vi "停止.vi"(6 "AxisHandle_Array":u32[](array[numeric]), 7 "索引":i32, 9 "停止模式":enum32{"Dec", "Emg"}(radio), 10 "reference输入":refnum<vi>, 11 "Boolean输入":refnum<vi>) -> (2 "急速停止成功":bool, 3 "减速停止成功":bool)   [LabVIEW 2016]
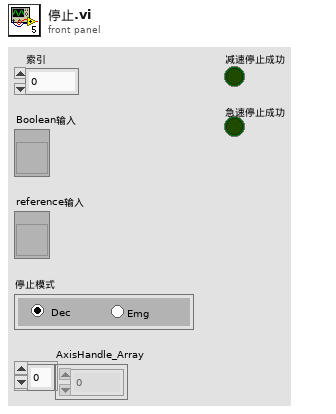
[diagram p1: front panel]
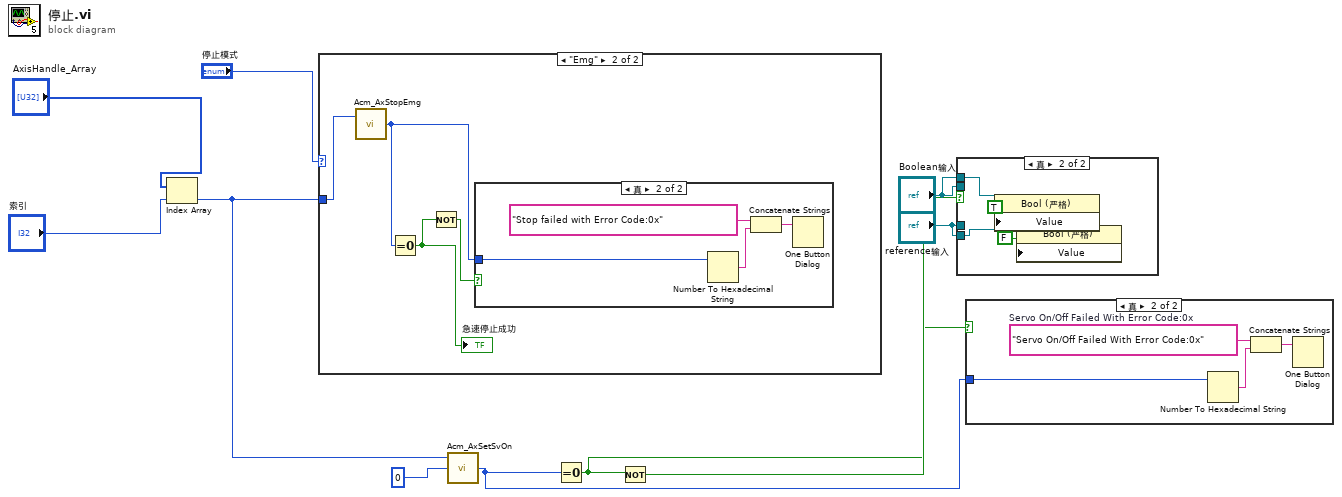
[diagram p0: block diagram]
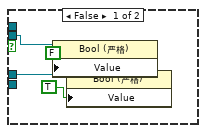
[diagram p2: hidden frame]
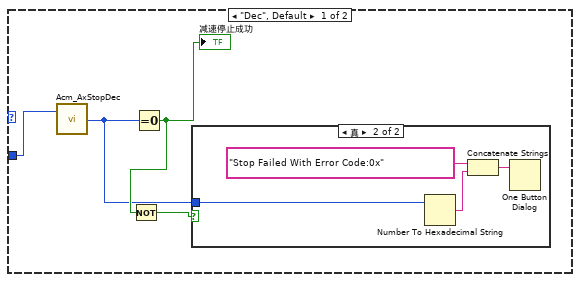
[diagram p4: hidden frame]
diagram:
  n1 = Index Array(array="AxisHandle_Array", index="索引") -> (element=w6:u32)
  n2 = case shown="\"Emg\"" "停止模式" {
    tunnel: w6 -> [w14 w22]
    frame "Dec", Default {
      n3 = call <userlib>:"Acm_AxStopDec.vi"("AxisHandle"=w14) -> ("ReturnValue"=w11:u32)  [unwired: 1 in, 2 out]
      n4 = Equal To 0?(x=w11) -> (x = 0?=w13:bool)
      "减速停止成功" <- w13
      n5 = Not(x=w13) -> (.not. x?=w12:bool)
      n6 = case shown="真" w12 {
        tunnel: w11 -> [_ w18]
        frame False {
        }
        frame True {
          n7 = Number To Hexadecimal String(2:w18) -> (0:w16:string)  [unwired: 1 out]
          n8 = Concatenate Strings("Stop Failed With Error Code:0x", w16) -> (w15:string)
          n9 = One Button Dialog(message=w15) -> ()  [unwired: 2 out]
        }
      }
    }
    frame "Emg" {
      n10 = call <userlib>:"Acm_AxStopEmg.vi"("AxisHandle"=w22) -> ("ReturnValue"=w21:u32)  [unwired: 1 in, 2 out]
      n11 = Equal To 0?(x=w21) -> (x = 0?=w20:bool)
      "急速停止成功" <- w20
      n12 = Not(x=w20) -> (.not. x?=w19:bool)
      n13 = case shown="真" w19 {
        tunnel: w21 -> [_ w26]
        frame False {
        }
        frame True {
          n14 = Number To Hexadecimal String(2:w26) -> (0:w24:string)  [unwired: 1 out]
          n15 = Concatenate Strings("Stop failed with Error Code:0x", w24) -> (w23:string)
          n16 = One Button Dialog(message=w23) -> ()  [unwired: 2 out]
        }
      }
    }
  }
  n17 = call <userlib>:"Acm_AxSetSvOn.vi"("OnOff"=u32 0, "AxisHandle"=w6) -> ("ReturnValue"=w8:u32)  [unwired: 1 in, 2 out]
  n18 = Equal To 0?(x=w8) -> (x = 0?=w9:bool)
  n19 = Not(x=w9) -> (.not. x?=w10:bool)
  n20 = case shown="真" w10 {
    tunnel: "Boolean输入" -> [w28 _]
    tunnel: "reference输入" -> [w27 _]
    tunnel: "Boolean输入" -> [_ w32]
    tunnel: "reference输入" -> [_ w31]
    frame False {
      n21 = property class="Bool (严格)"(reference=w28, "Value"=FALSE ("私服使能")) -> ()  [unwired: 1 in, 2 out]
      n22 = property class="Bool (严格)"(reference=w27, "Value"=TRUE ("私服使能关闭")) -> ()  [unwired: 1 in, 2 out]
    }
    frame True {
      n23 = property class="Bool (严格)"(reference=w32, "Value"=TRUE ("私服使能")) -> ()  [unwired: 1 in, 2 out]
      n24 = property class="Bool (严格)"(reference=w31, "Value"=FALSE ("私服使能关闭")) -> ()  [unwired: 1 in, 2 out]
    }
  }
  n25 = case shown="真" w9 {
    tunnel: w8 -> [_ w35]
    frame False {
    }
    frame True {
      w38 = "Servo On/Off Failed With Error Code:0x"  # Servo On/Off Failed With Error Code:0x
      n26 = Number To Hexadecimal String(2:w35) -> (0:w37:string)  [unwired: 1 out]
      n27 = Concatenate Strings(w38, w37) -> (w36:string)
      n28 = One Button Dialog(message=w36) -> ()  [unwired: 2 out]
    }
  }
